vi "vel1.vi"(0 "dx":dbl, 1 "dy":dbl, 2 "bias":dbl, 3 "Angle1":dbl(knob)=-45.83837436417874 scale=-90.0..90.0, 4 "Angle 2":dbl(knob)=-72.06882847083946 scale=-90.0..90.0, 5 "v":dbl, 7 "L 1":dbl(slide)=80.0 scale=0.0..200.0, 9 "L 2":dbl(slide)=80.0 scale=0.0..200.0) -> (14 "vq":dbl[](array[numeric]) format="%.2f", 15 "J-1":T1)   [LabVIEW 2024]
uses:
  <vilib>/Analysis/Matrix/Datatypes/RealMatrix.ctl
  <vilib>/Analysis/baseanly.llb/A x B.vi
  <vilib>/Analysis/baseanly.llb/A x Vector.vi
  <vilib>/Analysis/NI_AALBase.lvlib
  <vilib>/Analysis/NI_AALPro.lvlib
  <vilib>/Analysis/_algsub.llb/Real PseudoInverse Matrix.vi
  <vilib>/Analysis/Matrix/NI_Matrix.lvlib
panel:
  out "J":T1
  out "xdotydot":dbl[](array[numeric])
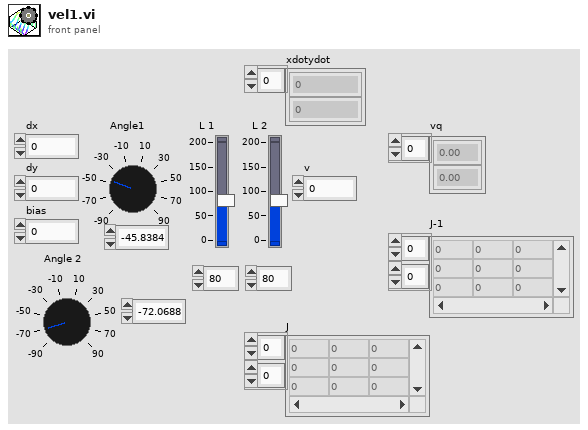
[diagram p1: front panel]
types:
  T1 = typedef "NI_Matrix.lvlib/RealMatrix.ctl" = dbl[][]
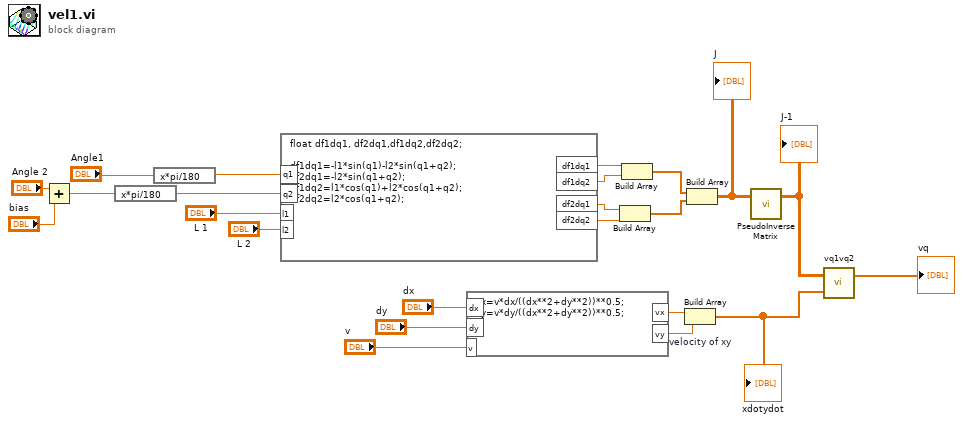
[diagram p0: block diagram]
diagram:
  n1 = Add(x="Angle 2", y="bias") -> (x+y=w6:dbl)
  n2 = expression code="x*pi/180"(w6) -> (w5:dbl)
  n3 = expression code="x*pi/180"("Angle1") -> (w4:dbl)
  n4 = formula code="float df1dq1, df2dq1,df1dq2,df2dq2;\n\ndf1dq1=-l1*sin(q1)-l2*sin(q1+q2);\ndf2dq1=-l2*sin(q1+q2);\ndf1dq2=l1*cos(q1)+l2*cos(q1+q2);\ndf2dq2=l2*cos(q1+q2);"("q1"=w4, "q2"=w5, "l1"="L 1", "l2"="L 2") -> ("df1dq1"=w19:dbl, "df1dq2"=w15:dbl, "df2dq1"=w14:dbl, "df2dq2"=w18:dbl)
  n5 = formula code="vx=v*dx/((dx**2+dy**2))**0.5;\nvy=v*dy/((dx**2+dy**2))**0.5;"("dx"="dx", "dy"="dy", "v"="v") -> ("vx"=w9:dbl, "vy"=w8:dbl)
  n6 = Build Array(w14, w18) -> (w16:dbl[])
  n7 = Build Array(w19, w15) -> (w17:dbl[])
  n8 = Build Array "velocity of xy"(w9, w8) -> (w13:dbl[])
  "xdotydot" <- w13
  n9 = Build Array(w17, w16) -> (w2:T1)
  "J" <- w2
  n10 = call-poly <vilib>:"PseudoInverse Matrix.vi"("Input Matrix"=w2) -> ("PseudoInverse Matrix"=w1:T1)  [unwired: 1 in, 1 out]
  "J-1" <- w1
  n11 = call-poly "vq1vq2"("Vector"=w13, "A"=w1) -> ("A x Vector"=→"vq":dbl[])  [unwired: 1 out]
